vi "StartAccelerometer.vi"(4 "Error In":errorcluster, 5 "Chip":enum16{"LSM6DS1", "LSM6DS3", "ADXL345"}(ring), 6 "I2C Channel (0)":u8, 7 "LINX Resource":T1) -> (0 "Error Out":errorcluster, 3 "LINX Resource":T1)   [LabVIEW 2015]
uses:
  <vilib>/LabVIEW Hacker/LINX/Private/Type Defs/LINX Ref.ctl
  <vilib>/LabVIEW Hacker/LINX/Private/Type Defs/Platform.ctl
  <vilib>/LabVIEW Hacker/LINX/Private/Type Defs/Interface.ctl
  <vilib>/LabVIEW Hacker/LINX/Private/Device/Type Defs/LINX Device Config.ctl
  <vilib>/LabVIEW Hacker/LINX/Private/Device/Type Defs/TCP Config.ctl
  <vilib>/LabVIEW Hacker/LINX/Private/Type Defs/Device Family.ctl
  <vilib>/LabVIEW Hacker/LINX/LVH-LINX.lvlib
  <vilib>/LabVIEW Hacker/LINX/Private/Device/Device.lvlib
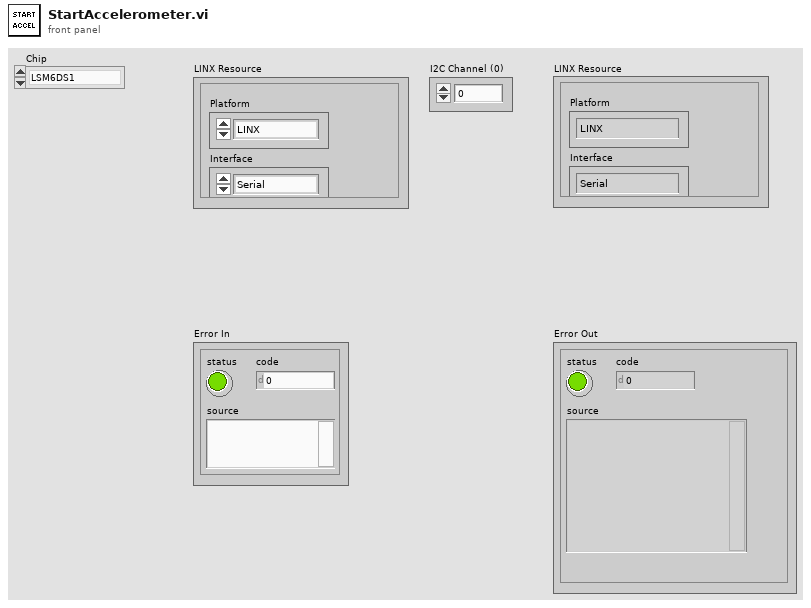
[diagram p1: front panel]
types:
  T1 = typedef "LVH-LINX.lvlib/LINX Ref.ctl" = cluster{"Platform":T2, "Interface":T3, "LINX Device Config":T4}
  T2 = typedef "LVH-LINX.lvlib/Platform.ctl" = enum16{"LINX", "myRIO"}
  T3 = typedef "LVH-LINX.lvlib/Interface.ctl" = enum16{"Serial", "TCP"}
  T4 = typedef "LVH-LINX.lvlib/Device.lvlib/LINX Device Config.ctl" = cluster{"Interface":T3, "COM Port":refnum<visa-resource-name>, "TCP Configuration":T5, "Device Family":T6, "Device ID":u8, "Device Name":string, "TCP Ref":refnum<k5>}
  T5 = typedef "LVH-LINX.lvlib/Device.lvlib/TCP Config.ctl" = cluster{"IP Address":string, "Port":u16}
  T6 = typedef "LVH-LINX.lvlib/Device Family.ctl" = enum8{"National Instruments", "Digilent", "Arduino"}
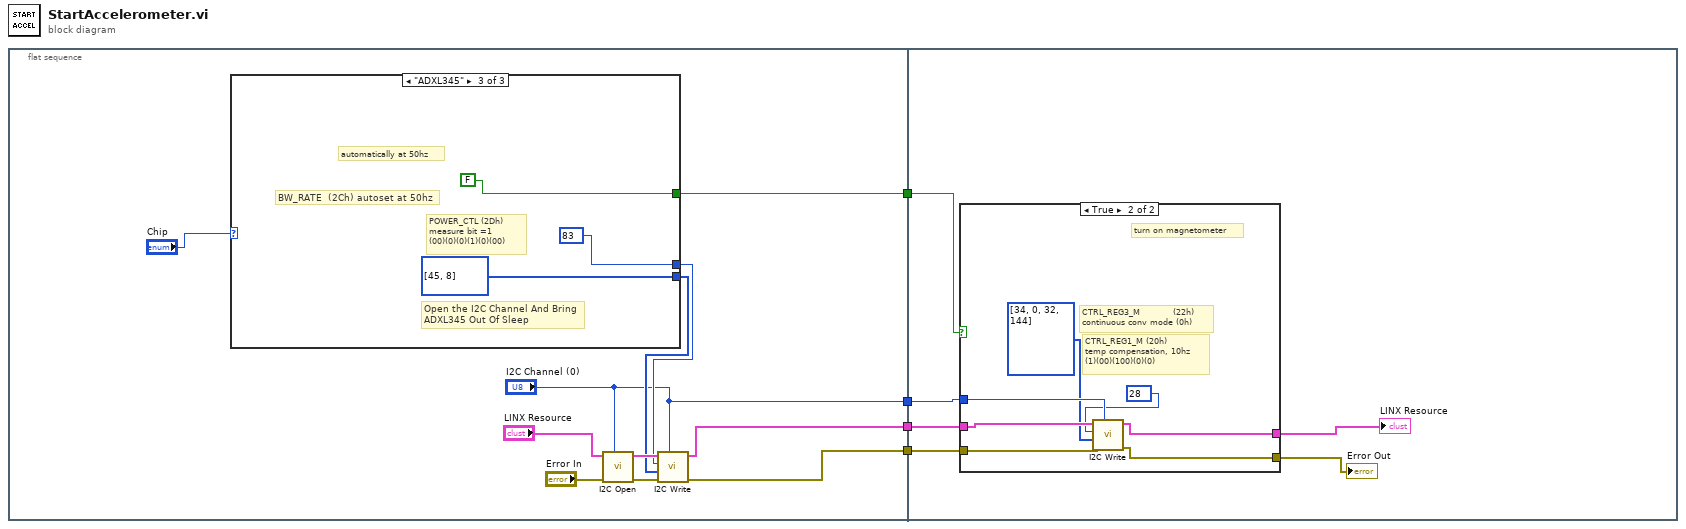
[diagram p0: block diagram]
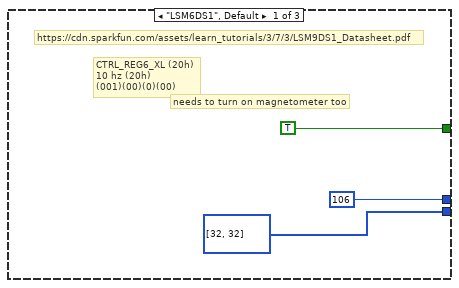
[diagram p2: hidden frame]
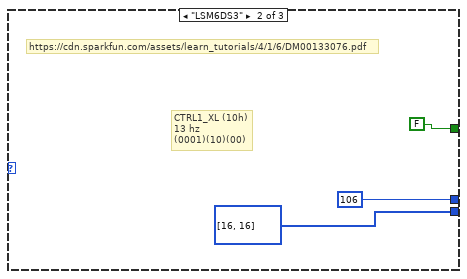
[diagram p3: hidden frame]
diagram:
  n1 = flat-sequence {
    tunnel: [w8] -> w4
    tunnel: [w7] -> w3
    tunnel: [w6] -> w2
    tunnel: ["I2C Channel (0)"] -> w1
    tunnel: w4 -> [w30]
    tunnel: w3 -> [w29]
    tunnel: w2 -> [w27]
    tunnel: w1 -> [w25]
    frame #0 {
      n2 = case shown="\"ADXL345\"" "Chip" {
        tunnel: [u8[] [32, 32] ("Data") u8[] [16, 16] ("Data") u8[] [45, 8] ("Data")] -> w12
        tunnel: [u8 106 ("I2C Slave Address (0)") u8 106 ("I2C Slave Address (0)") u8 83 ("I2C Slave Address (0)")] -> w11
        tunnel: [TRUE FALSE FALSE] -> w8
        frame "LSM6DS1", Default {
          # "https://cdn.sparkfun.com/assets/learn_tutorials/3/7/3/LSM9DS1_Datasheet.pdf"
          # "CTRL_REG6_XL (20h)\n10 hz (20h)\n(001)(00)(0)(00)"
          # "needs to turn on magnetometer too"
        }
        frame "LSM6DS3" {
          # "https://cdn.sparkfun.com/assets/learn_tutorials/4/1/6/DM00133076.pdf"
          # "CTRL1_XL (10h)\n13 hz \n(0001)(10)(00)"
        }
        frame "ADXL345" {
          # "BW_RATE  (2Ch) autoset at 50hz"
          # "automatically at 50hz"
          # "POWER_CTL (2Dh)\nmeasure bit =1\n(00)(0)(0)(1)(0)(00)"
          # "Open the I2C Channel And Bring \nADXL345 Out Of Sleep"
        }
      }
      n3 = call <vilib>:"I2C Open.vi"("I2C Channel (0)"="I2C Channel (0)", "Error In"="Error In", "LINX Resource"="LINX Resource") -> ("Error Out"=w13:errorcluster, "LINX Resource"=w14:T1)  [unwired: 7 in]
      n4 = call <vilib>:"I2C Write.vi"("I2C Channel"="I2C Channel (0)", "Error In"=w13, "Data"=w12, "I2C Slave Address (0)"=w11, "LINX Resource"=w14) -> ("Error Out"=w6:errorcluster, "LINX Resource"=w7:T1)  [unwired: 5 in]
    }
    frame #1 {
      n5 = case shown="True" w30 {
        tunnel: w29 -> [w32 w39]
        tunnel: [w32 w36] -> w28
        tunnel: [w31 w35] -> w26
        tunnel: w27 -> [w31 w38]
        tunnel: w25 -> [_ w37]
        frame False {
          # "dont need to turn on magnetometer"
        }
        frame True {
          # "CTRL_REG1_M (20h)\ntemp compensation, 10hz\n(1)(00)(100)(0)(0)"
          # "CTRL_REG3_M           (22h)\ncontinuous conv mode (0h)"
          # "turn on magnetometer"
          n6 = call <vilib>:"I2C Write.vi"("I2C Channel"=w37, "Error In"=w38, "Data"=u8[] [34, 0, 32, 144], "I2C Slave Address (0)"=u8 28, "LINX Resource"=w39) -> ("Error Out"=w35:errorcluster, "LINX Resource"=w36:T1)  [unwired: 5 in]
        }
      }
      "LINX Resource" <- w28
      "Error Out" <- w26
    }
  }
